vi "PicoScope5000aGetTimebase2.vi"(4 "Number of Samples":u32, 6 "Memory Segment":u32, 7 "Acquisition Settings":T2={"preTriggerSamples"=0, "postTriggerSamples"=1000, "timebase"=2} {"postTriggerSamples" format="%_6p"; "preTriggerSamples" format="%_6p"}, 10 "handle in":i16, 11 "error in (no error)":errorcluster) -> (2 "handle out":i16, 3 "error out":errorcluster, 5 "Properties Panel":T1 {"Max Total Capture Time Available (sec)" format="%.3p"; "Sample Frequency" format="%.3p"; "Sample Rate" format="%.3p"; "Max Samples Available" format="%.3p"; "Total Capture Time (sec)" format="%.3p"})   [LabVIEW 2020]
uses:
  shared/Acquisition Settings.ctl
  ps5000a.dll
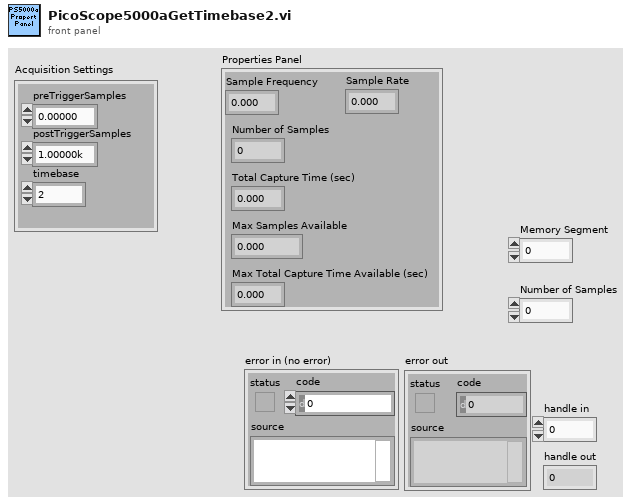
[diagram p1: front panel]
types:
  T1 = cluster{"Sample Frequency":sgl, "Sample Rate":sgl, "Max Samples Available":i32, "Number of Samples":u32, "Total Capture Time (sec) ":sgl, "Max Total Capture Time Available (sec)":sgl}
  T2 = typedef "Acquisition Settings.ctl" = cluster{"preTriggerSamples":u64, "postTriggerSamples":u64, "timebase":u32}
  T3 = cluster{sgl, sgl, "maxSamples":i32, "Number of Samples":u32, sgl, sgl}
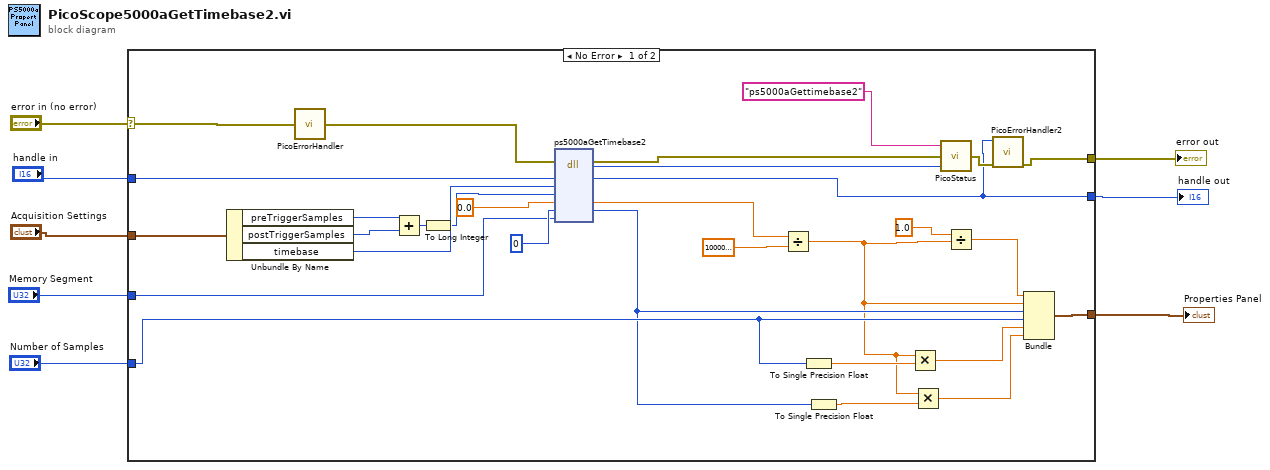
[diagram p0: block diagram]
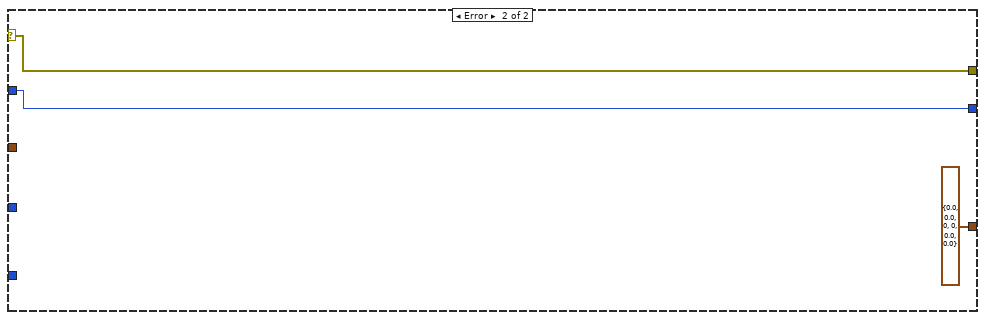
[diagram p2: hidden frame]
diagram:
  n1 = case shown="No Error" "error in (no error)" {
    selector: "error in (no error)" -> [w28 w41]
    tunnel: [w13 w41] -> w8
    tunnel: [w11 w40] -> w7
    tunnel: "Memory Segment" -> [w27 _]
    tunnel: "Number of Samples" -> [w22 _]
    tunnel: "handle in" -> [w26 w40]
    tunnel: "Acquisition Settings" -> [w25 _]
    tunnel: [w18 T3 {0.0, 0.0, "maxSamples"=0, "Number of Samples"=0, 0.0, 0.0}] -> w1
    frame No Error {
      n2 = Unbundle By Name(w25) -> ("preTriggerSamples"=w32:u64, "postTriggerSamples"=w33:u64, "timebase"=w34:u32)
      n3 = call "PicoErrorHandler.vi"("error in"=w28) -> ("error out"=w36:errorcluster)
      n4 = Add(x=w32, y=w33) -> (x+y=w10:u64)
      n5 = To Long Integer(number=w10) -> (32bit integer=w9:i32)
      n6 = dll-call lib="ps5000a.dll" fn="ps5000aGetTimebase2"(error in=w36, "handle"=w26, "timebase"=w34, "noSamples"=w9, "timeIntervalNanoseconds"=sgl 0.0, "maxSamples"=0, "segmentIndex"=w27) -> (error out=w35:errorcluster, "PICO_STATUS"=w12:u32, "handle"=w11:i16, "timeIntervalNanoseconds"=w37:sgl, "maxSamples"=w20:i32)  [unwired: 5 in, 1 out]
      n7 = Divide(x=w37, y=sgl 1000000000.0) -> (x/y=w17:sgl)
      n8 = To Single Precision Float(number=w22) -> (single precision float=w24:sgl)
      n9 = To Single Precision Float(number=w20) -> (single precision float=w21:sgl)
      n10 = Multiply(x=w17, y=w24) -> (x*y=w23:sgl)
      n11 = Multiply(x=w17, y=w21) -> (x*y=w19:sgl)
      n12 = call "PicoStatus.vi"("PICO STATUS"=w12, "error in"=w35, "source"="ps5000aGettimebase2") -> ("error out"=w14:errorcluster)
      n13 = Divide(x=sgl 1.0, y=w17) -> (x/y=w15:sgl)
      n14 = call "PicoErrorHandler2.vi"("error in (no error)"=w14, "handle In"=w11) -> ("error out"=w13:errorcluster)  [unwired: 9 in]
      n15 = Bundle(w15, w17, "maxSamples"=w20, "Number of Samples"=w22, w23, w19) -> (w18:T3)  [unwired: 1 in]
    }
    frame Error {
    }
  }
  "error out" <- w8
  "handle out" <- w7
  "Properties Panel" <- w1
